vi "EvaluateExpression.vi"(11 "Parsed Expression":T1={"String"="", "avgs"=[{"Expression"="", "Durration"=0.0, "Replacement"="", "Values"=[]}]}) -> (0 "error out":errorcluster, 2 "Result":dbl)   [LabVIEW 2012]
panel:
  in  "error in (no error)":errorcluster
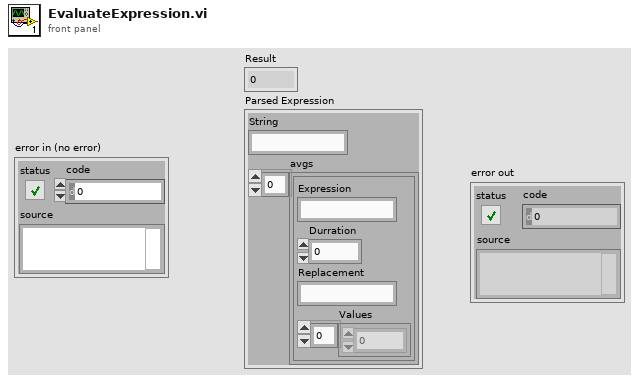
[diagram p1: front panel]
types:
  T1 = cluster{"String":string, "avgs":cluster{"Expression":string, "Durration":dbl, "Replacement":string, "Values":dbl[]}[]}
  T2 = cluster{"parameter name":string, "parameter content":string}
  T3 = cluster{"Expression":string, "Durration":dbl, "Replacement":string, "Values":dbl[]}[]
  T4 = cluster{"parameter name":string, "parameter content":string}[]
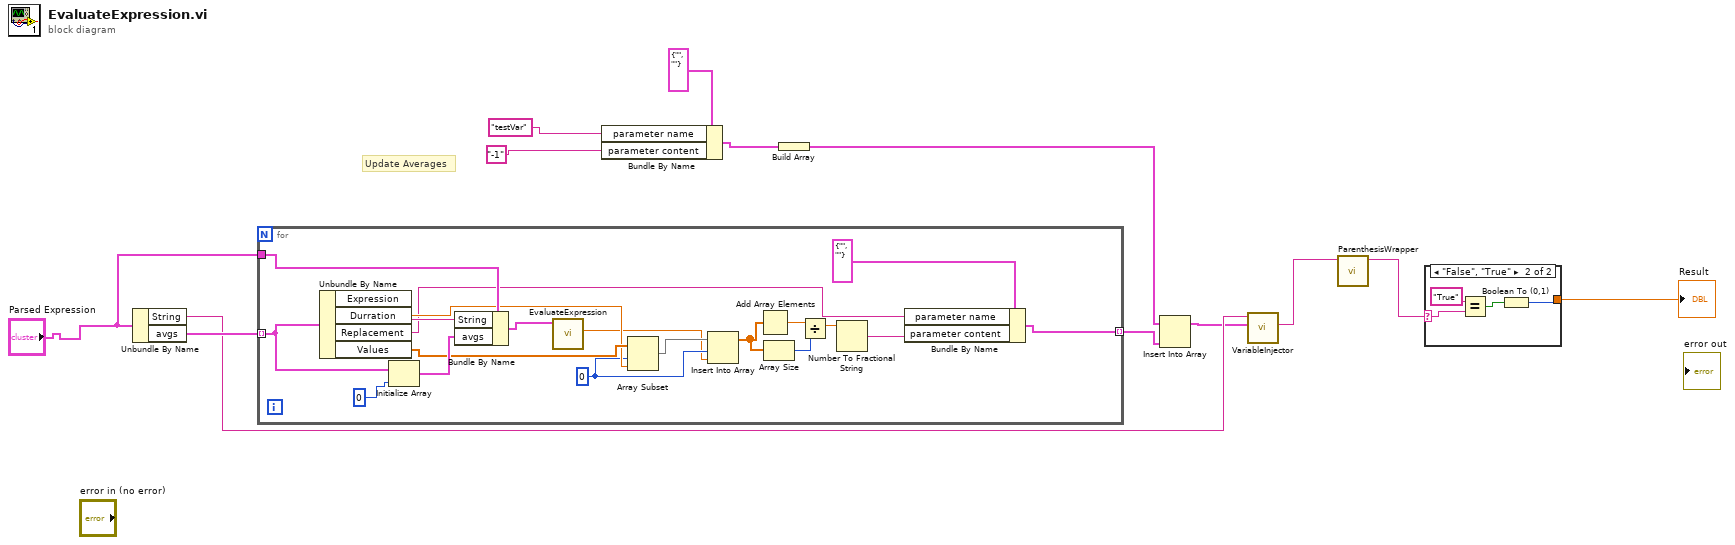
[diagram p0: block diagram]
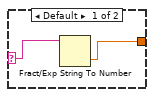
[diagram p2: hidden frame]
diagram:
  # "Update Averages"
  n1 = Unbundle By Name("Parsed Expression") -> ("String"=w2:string, "avgs"=w13:T3)
  n2 = for {
    tunnel: w13 -> [w29] mode=indexing
    tunnel: "Parsed Expression" -> [w32]
    tunnel: [w14] -> w11 mode=indexing
    w24 = 0
    n3 = Unbundle By Name(w29) -> ("Expression"=w31:string, "Durration"=w25:dbl, "Replacement"=w17:string, "Values"=w26:dbl[])
    n4 = Initialize Array(w29, 0) -> (w28:T3)
    n5 = Bundle By Name(cluster=w32, "String"=w31, "avgs"=w28) -> (w27:T1)
    n6 = call "EvaluateExpression.vi"("Parsed Expression"=w27) -> ("Result"=w22:dbl)  [unwired: 9 in, 1 out]
    n7 = Array Subset(array=w26, index=w24, length=w25) -> (w23:dbl[])
    n8 = Insert Into Array(array=w23, index=w24, new element=w22) -> (w21:dbl[])
    n9 = Add Array Elements(numeric array=w21) -> (sum=w20:dbl)
    n10 = Array Size(array=w21) -> (size(s)=w19:i32)
    n11 = Divide(x=w20, y=w19) -> (x/y=w16:dbl)
    n12 = Number To Fractional String(number=w16) -> (F-format string=w15:string)  [unwired: 3 in]
    n13 = Bundle By Name(cluster=T2 {"parameter name"="", "parameter content"=""}, "parameter name"=w17, "parameter content"=w15) -> (w14:T2)
  }
  n14 = Bundle By Name(cluster=T2 {"parameter name"="", "parameter content"=""}, "parameter name"="testVar", "parameter content"="-1") -> (w8:T2)
  n15 = Build Array(w8) -> (w10:T4)
  n16 = Insert Into Array(array=w10, new element=w11) -> (w1:T4)  [unwired: 1 in]
  n17 = call "VariableInjector.vi"("Variables"=w1, "Expression"=w2) -> ("Result"=w5:string)  [unwired: 9 in]
  n18 = call "ParenthesisWrapper.vi"("Input"=w5) -> ("Output"=w4:string)  [unwired: 10 in]
  n19 = case shown="\"False\", \"True\"" w4 {
    selector: w4 -> [w34 w37]
    tunnel: [w33 w35] -> w3
    frame Default {
      n20 = Fract/Exp String To Number(string=w34) -> (number=w33:dbl)  [unwired: 3 in, 1 out]
    }
    frame "False", "True" {
      n21 = Equal?(x="True", y=w37) -> (x = y?=w36:bool)
      n22 = Boolean To (0,1)(Boolean=w36) -> (0, 1=w35:i16)
    }
  }
  "Result" <- w3
